vi "FGV T90.vi"(0 "Gas Konfig":T1={"Gasflasche"=0, "Konfig Gasflasche"=FALSE, "Auswahl"=0, "Sollwert"=0.0, "Abweichung"=0.0, "max. Responsetime"=0.0, "Modus:"=0, "Abschaltzeit"=1.0, "Stabilisierungszeit"=1.0, "Bearbeiter"=""} {"Stabilisierungszeit" format="%#_5g"; "Abschaltzeit" format="%#_5g"; "Modus:" items=["Cal Gas", "Entnahmestelle"]; "max. Responsetime" format="%#_5g"; "Abweichung" format="%#_5g"; "Sollwert" format="%#_5g"; "Gasflasche" items=["----"=10000, "IAG NH3 3000"=0, "IAG NH3 200"=1, "IAG NH3 2000"=2, "IAG MG"=3, "IAG O2"=4]}, 2 "Protokolldaten":cluster{"File Name":T7, "Pfad:":T8}, 4 "aktiv":bool, 6 "Zustand":T9, 9 "Entnahme aktiv":bool, 10 "Overflow Leak":bool, 11 "error in (no error)":errorcluster caption="Fehler (Eingang, kein Fehler)", 13 "Aktion":T10) -> (14 "Overflow Leak":bool, 15 "error out":errorcluster caption="Fehler (Ausgang)", 17 "Entnahme aktiv":bool, 20 "Gas Konfig":T1={"Gasflasche"=0, "Konfig Gasflasche"=FALSE, "Auswahl"=0, "Sollwert"=0.0, "Abweichung"=0.0, "max. Responsetime"=0.0, "Modus:"=1, "Abschaltzeit"=0.0, "Stabilisierungszeit"=1.0, "Bearbeiter"=""} {"Stabilisierungszeit" format="%#_5g"; "Abschaltzeit" format="%#_5g"; "Modus:" items=["Cal Gas", "Entnahmestelle"]; "max. Responsetime" format="%#_5g"; "Abweichung" format="%#_5g"; "Sollwert" format="%#_5g"; "Gasflasche" items=["----"=10000, "IAG NH3 3000"=0, "IAG NH3 200"=1, "IAG NH3 2000"=2, "IAG MG"=3, "IAG O2"=4]}, 22 "Protokolldaten":cluster{"File Name":T7, "Pfad":T8}, 24 "aktiv":bool, 26 "Zustand":T9)   [LabVIEW 2020, in "T90.lvlib"]
uses:
  T90.lvlib
  Aktion FGV T90.ctl
  Aktion Zustandsautomat.ctl
  Visualisierungs Elemente/String - Eingabefeld.ctl
  Visualisierungs Elemente/Pfad-Eingabefeld.ctl
  T90 Gas Konfig.ctl
  Seiten/System Einstellungen V2/Gasflasche Auswahl.ctl
  Seiten/System Einstellungen V2/Konfig Gasflasche.ctl
  Visualisierungs Elemente/Auswahlfeld.ctl
  Visualisierungs Elemente/Zahlen-Eingabefeld.ctl
  Zustand Auswahl.ctl
  Allgemein/allgemeine Sub-VIs.lvlib
  Seiten/System Einstellungen V2/System Einstellungen V2.lvlib
panel:
  # "File Name:"
  # "Pfad:"
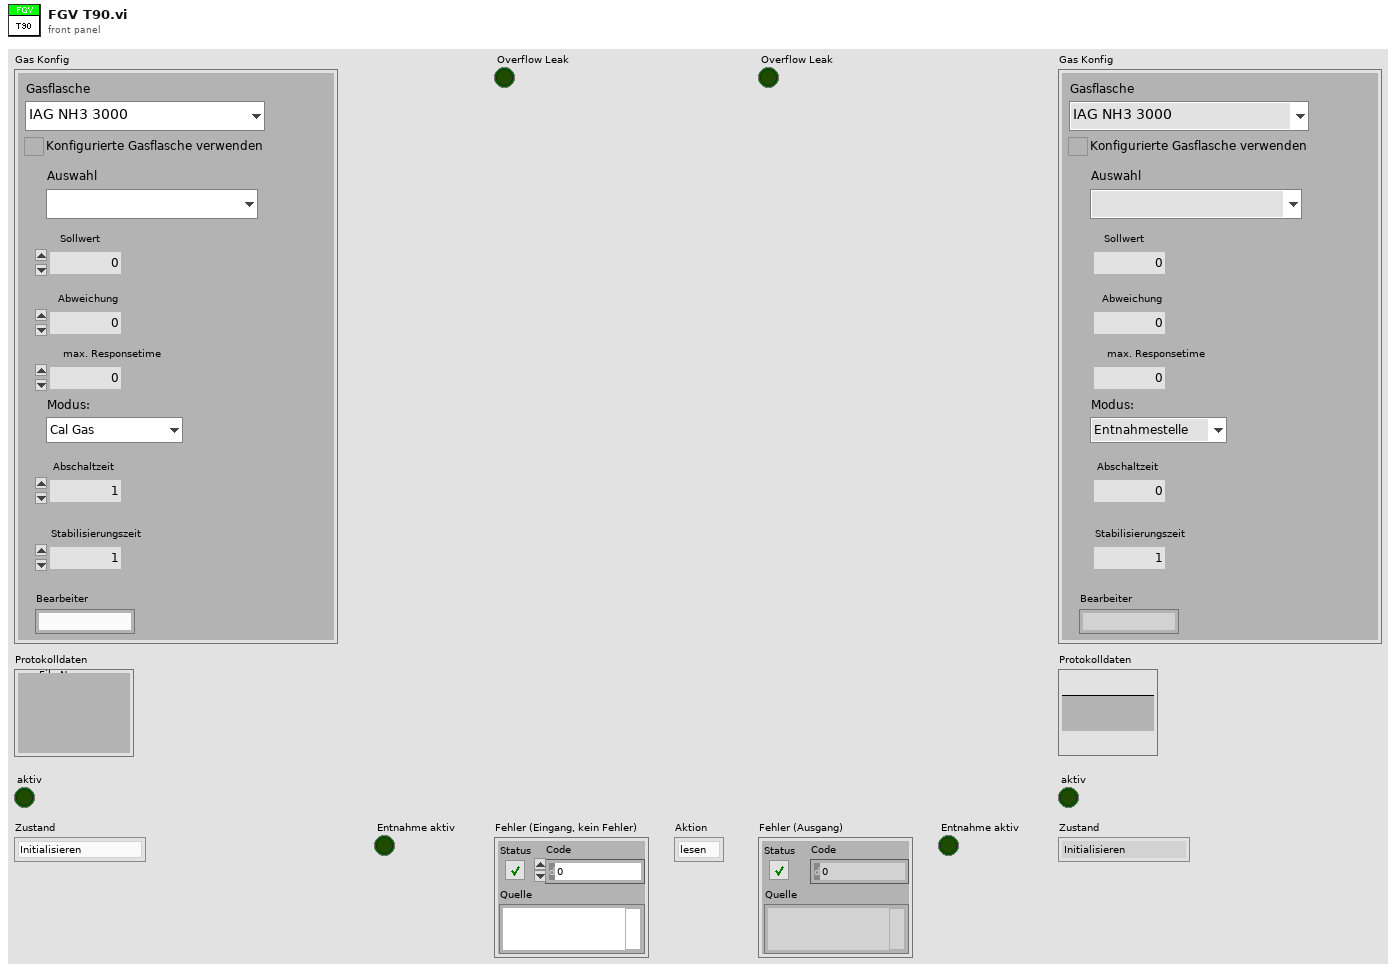
[diagram p1: front panel]
types:
  T1 = typedef "T90.lvlib/T90 Gas Konfig.ctl" = cluster{"Gasflasche":T2, "Konfig Gasflasche":T3, "Auswahl":T4, "Sollwert":T5, "Abweichung":T5, "max. Responsetime":T5, "Modus:":T6, "Abschaltzeit":T5, "Stabilisierungszeit":T5, "Bearbeiter":string}
  T2 = typedef "System Einstellungen V2.lvlib/Gasflasche Auswahl.ctl" = u16
  T3 = typedef "System Einstellungen V2.lvlib/Konfig Gasflasche.ctl" = bool
  T4 = typedef "Auswahlfeld.ctl" = u16
  T5 = typedef "Zahlen-Eingabefeld.ctl" = sgl
  T6 = typedef "T90.lvlib/Zustand Auswahl.ctl" = u16
  T7 = typedef "String - Eingabefeld.ctl" = string
  T8 = typedef "Pfad-Eingabefeld.ctl" = path
  T9 = typedef "T90.lvlib/Aktion Zustandsautomat.ctl" = enum16{"Initialisieren", "Warten", "Gas aufschalten", "Stabilisieren", "Volle Konzentration 1", "Berechnen", "Prüfung starten", "Prüfung", "Prüfung beenden", "keine Funktion"}
  T10 = typedef "T90.lvlib/Aktion FGV T90.ctl" = enum16{"lesen", "schreiben", "laden", "speichern", "T90 aktiv", "T90 Entnahme aktiv", "Overflow Leak", "Pfad", "Zustand", "max. Responsetime"}
  T11 = cluster{"Gas Konfig":T1, "File Name":T7, "Pfad:":T8}
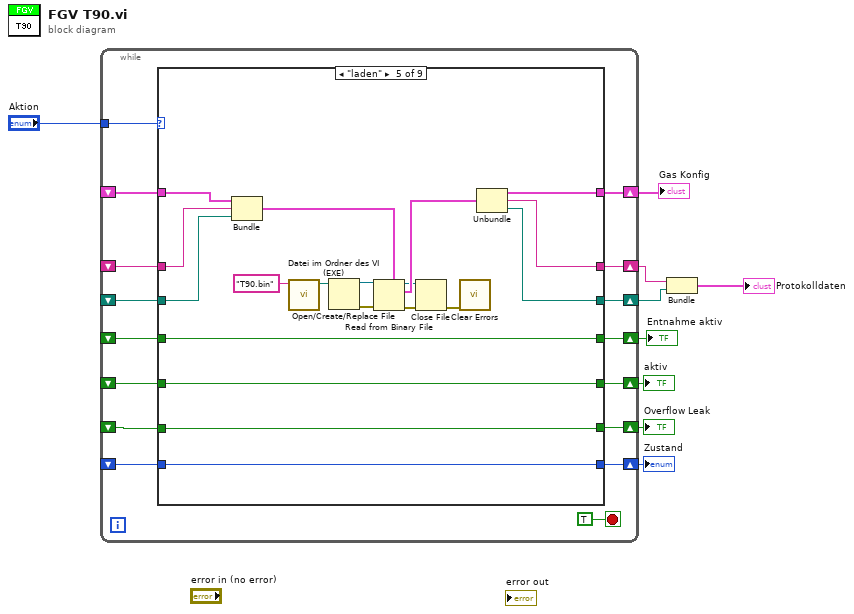
[diagram p0: block diagram]
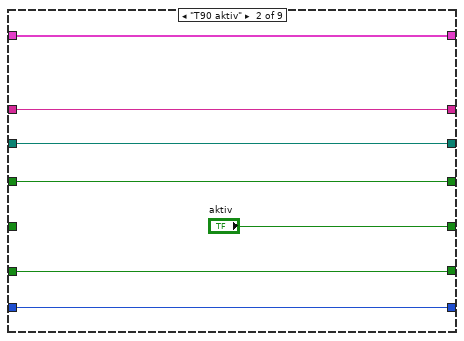
[diagram p3: hidden frame]
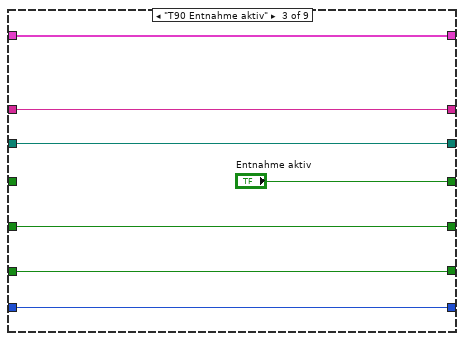
[diagram p4: hidden frame]
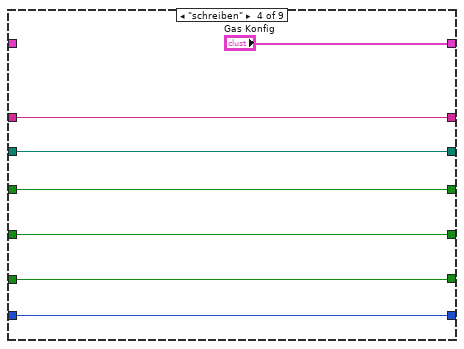
[diagram p5: hidden frame]
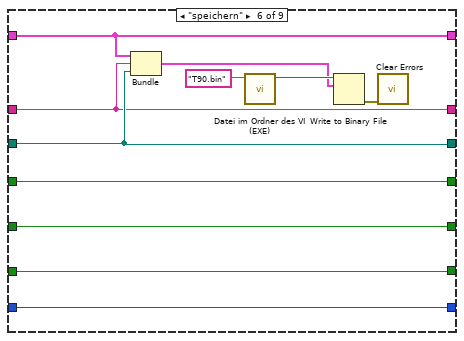
[diagram p6: hidden frame]
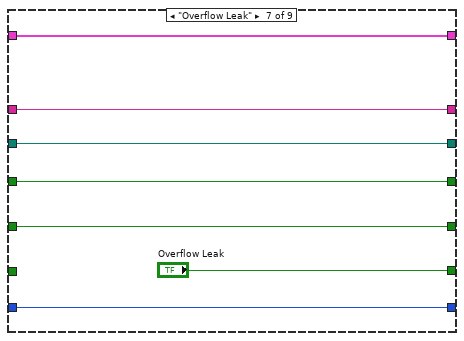
[diagram p7: hidden frame]
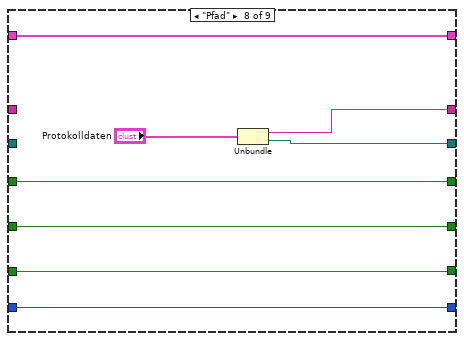
[diagram p8: hidden frame]
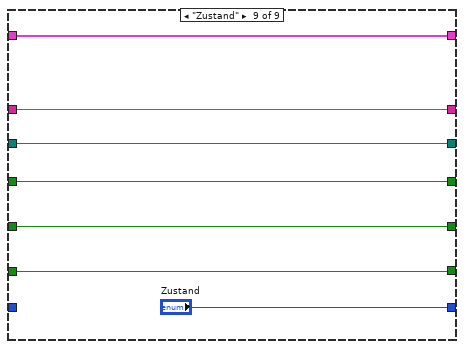
[diagram p9: hidden frame]
diagram:
  n1 = while {
    tunnel: "Aktion" -> [w24]
    shift-right: [w23] -> w1
    shift-left: _ -> [w22]
    shift-right: [w21] -> w8
    shift-left: _ -> [w20]
    shift-right: [w19] -> w7
    shift-left: _ -> [w18]
    shift-right: [w17] -> w4
    shift-left: _ -> [w16]
    shift-right: [w15] -> w3
    shift-left: _ -> [w14]
    shift-right: [w13] -> w6
    shift-left: _ -> [w12]
    shift-right: [w11] -> w5
    shift-left: _ -> [w10]
    stop <- TRUE stop-if-true
    n2 = case shown="\"laden\"" w24 {
      tunnel: [w32 w39 w45 "Gas Konfig" w56 w81 w89 w96 w99] -> w23
      tunnel: w22 -> [w32 w39 w45 _ w71 w81 w89 w96 w99]
      tunnel: [w31 "aktiv" w44 w53 w68 w78 w86 w95 w102] -> w21
      tunnel: w20 -> [w31 _ w44 w53 w68 w78 w86 w95 w102]
      tunnel: [w30 w37 "Entnahme aktiv" w52 w67 w77 w90 w98 w105] -> w19
      tunnel: w18 -> [w30 w37 _ w52 w67 w77 w90 w98 w105]
      tunnel: [w28 w36 w43 w50 w55 w75 w88 w92 w100] -> w17
      tunnel: w16 -> [w28 w36 w43 w50 w65 w75 w88 _ w100]
      tunnel: [w29 w35 w42 w49 w54 w76 w87 w91 w101] -> w15
      tunnel: w14 -> [w29 w35 w42 w49 w64 w76 w87 _ w101]
      tunnel: [w27 w34 w41 w51 w66 w74 "Overflow Leak" w97 w104] -> w13
      tunnel: w12 -> [w27 w34 w41 w51 w66 w74 _ w97 w104]
      tunnel: [w26 w33 w40 w48 w63 w73 w84 w94 "Zustand"] -> w11
      tunnel: w10 -> [w26 w33 w40 w48 w63 w73 w84 w94 _]
      frame "lesen", Default {
      }
      frame "T90 aktiv" {
      }
      frame "T90 Entnahme aktiv" {
      }
      frame "schreiben" {
      }
      frame "laden" {
        n3 = Bundle("Gas Konfig"=w71, "File Name"=w65, "Pfad:"=w64) -> (w70:T11)  [unwired: 1 in]
        n4 = call "Datei im Ordner des VI (EXE).vi"("Dateiname"="T90.bin") -> ("Dateipfad im Ordner des Haupt-VIs"=w62:path)  [unwired: 8 in, 2 out]
        n5 = Open/Create/Replace File(file path (use dialog)=w62) -> (refnum out=w61:refnum<file>, error out=w60:errorcluster)  [unwired: 5 in, 1 out]
        n6 = Read from Binary File(5:w70, 8:w60, 11:w61) -> (0:w59:errorcluster, 2:w69:T11, 3:w58:refnum<file>)  [unwired: 3 in, 1 out]
        n7 = Close File(refnum=w58, error in=w59) -> (error out=w57:errorcluster)  [unwired: 1 out]
        n8 = call <vilib>:"Clear Errors.vi"("error in (no error)"=w57) -> ()  [unwired: 5 in, 2 out]
        n9 = Unbundle(w69) -> ("Gas Konfig"=w56:T1, "File Name"=w55:T7, "Pfad:"=w54:T8)
      }
      frame "speichern" {
        n10 = Bundle("Gas Konfig"=w81, "File Name"=w75, "Pfad:"=w76) -> (w80:T11)  [unwired: 1 in]
        n11 = call "Datei im Ordner des VI (EXE).vi"("Dateiname"="T90.bin") -> ("Dateipfad im Ordner des Haupt-VIs"=w82:path)  [unwired: 8 in, 2 out]
        n12 = Write to Binary File(file (use dialog)=w82, data=w80) -> (error out=w79:errorcluster)  [unwired: 4 in, 2 out]
        n13 = call <vilib>:"Clear Errors.vi"("error in (no error)"=w79) -> ()  [unwired: 5 in, 2 out]
      }
      frame "Overflow Leak" {
      }
      frame "Pfad" {
        n14 = Unbundle("Protokolldaten") -> ("File Name"=w92:T7, "Pfad:"=w91:T8)
      }
      frame "Zustand" {
      }
    }
  }
  "aktiv" <- w8
  "Entnahme aktiv" <- w7
  "Overflow Leak" <- w6
  "Zustand" <- w5
  "Gas Konfig" <- w1
  n15 = Bundle("File Name"=w4, "Pfad:"=w3) -> (→"Protokolldaten":cluster{"File Name":T7, "Pfad:":T8})  [unwired: 1 in]
